vi "Test Add Parent UID To Child Node.vi"(8 "error in (no error)":errorcluster) -> (0 "error out":errorcluster)   [LabVIEW 2017, in "Unit Tests.lvlib"]
uses:
  Unit Tests.lvlib
  source/Browser Core/Server Classes/Base Tree/Base Tree.lvclass
  source/Browser Core/Node Classes/Generic Node/Generic Node.lvclass
  source/Browser Core/Server Classes/Base Tree/Base Tree.lvclass/Base Tree.ctl
  source/Browser Core/Node Classes/Generic Node/Generic Node.lvclass/Generic Node.ctl
  <vilib>/addons/_JKI Toolkits/Caraya/classes/Test/Test.lvclass
  <vilib>/addons/_JKI Toolkits/Caraya/classes/Assert/Assert.lvclass
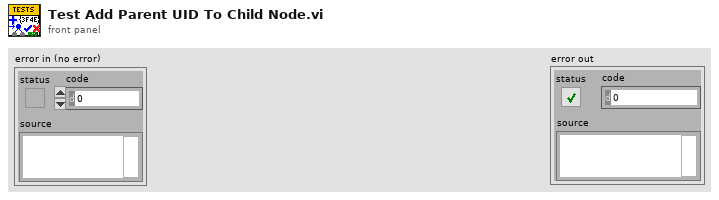
[diagram p1: front panel]
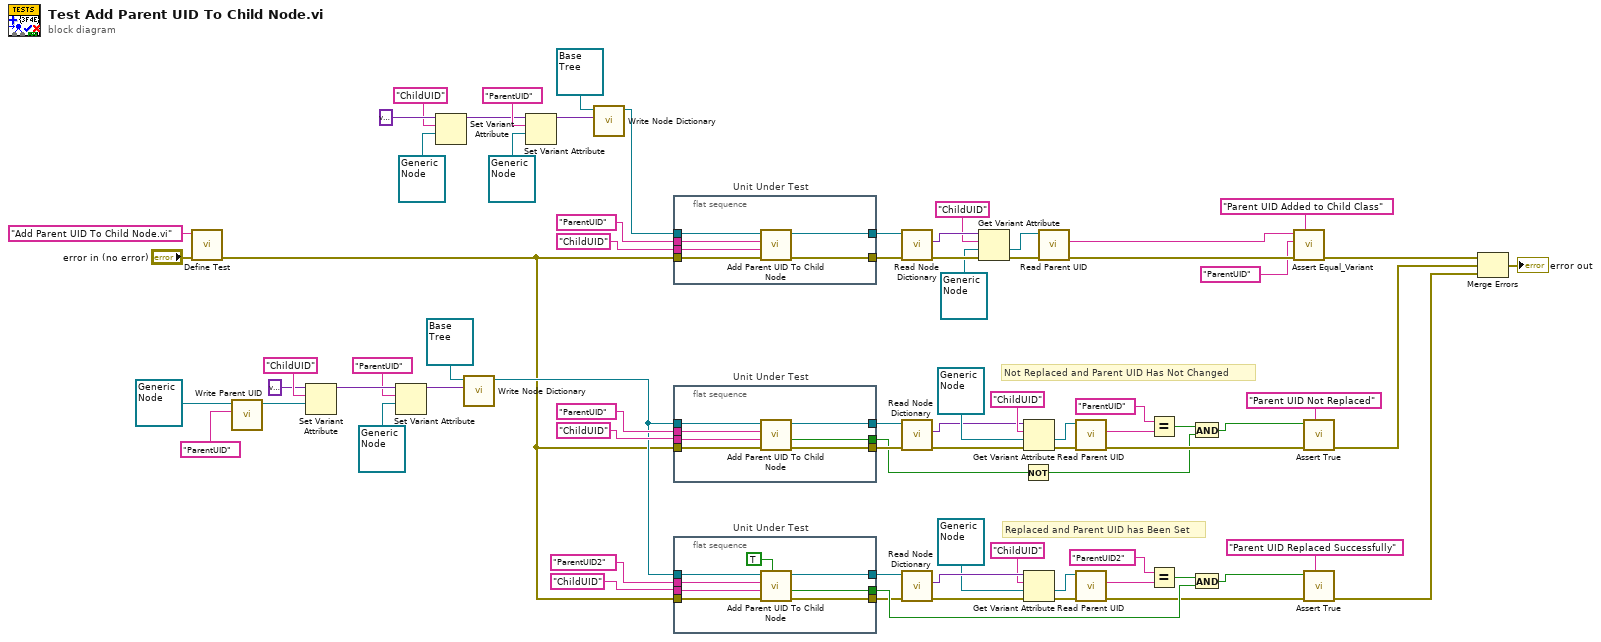
[diagram p0: block diagram]
diagram:
  # "Replaced and Parent UID has Been Set"
  # "Not Replaced and Parent UID Has Not Changed"
  n1 = call <vilib>:"Define Test.vi"("error in (no error)"="error in (no error)", "Label (VI Title)"="Add Parent UID To Child Node.vi") -> ("error out"=w3:errorcluster)  [unwired: 9 in]
  n2 = call "Write Parent UID.vi"("Parent UID"="ParentUID" ("name"), "Generic Node in"=refnum<class "Generic Node.lvclass"> refnum ("Browser Core.lvlib:Generic Node.lvclass")) -> ("Generic Node out"=w28:refnum<class "Generic Node.lvclass">)  [unwired: 8 in, 1 out]
  n3 = Set Variant Attribute(Variant=variant ("variant"), name="ChildUID", value=w28) -> (Variant out=w36:variant)  [unwired: 1 in, 2 out]
  n4 = Set Variant Attribute(Variant=w36, name="ParentUID", value=refnum<class "Generic Node.lvclass"> refnum ("Browser Core.lvlib:Generic Node.lvclass")) -> (Variant out=w37:variant)  [unwired: 1 in, 2 out]
  n5 = Set Variant Attribute(Variant=variant ("variant"), name="ChildUID", value=refnum<class "Generic Node.lvclass"> refnum ("Browser Core.lvlib:Generic Node.lvclass")) -> (Variant out=w68:variant)  [unwired: 1 in, 2 out]
  n6 = call "Write Node Dictionary.vi"("Node Dictionary"=w37, "Base Tree in"=refnum<class "Base Tree.lvclass"> refnum) -> ("Base Tree out"=w4:refnum<class "Base Tree.lvclass">)  [unwired: 8 in, 1 out]
  n7 = Set Variant Attribute(Variant=w68, name="ParentUID", value=refnum<class "Generic Node.lvclass"> refnum ("Browser Core.lvlib:Generic Node.lvclass")) -> (Variant out=w67:variant)  [unwired: 1 in, 2 out]
  n8 = call "Write Node Dictionary.vi"("Node Dictionary"=w67, "Base Tree in"=refnum<class "Base Tree.lvclass"> refnum) -> ("Base Tree out"=w40:refnum<class "Base Tree.lvclass">)  [unwired: 8 in, 1 out]
  n9 = flat-sequence "Unit Under Test" {
    tunnel: w3 -> [w82]
    tunnel: w40 -> [w81]
    tunnel: "ParentUID" ("name") -> [w80]
    tunnel: "ChildUID" ("name") -> [w79]
    tunnel: [w78] -> w64
    tunnel: [w77] -> w63
    frame #0 {
      n10 = call "Add Parent UID To Child Node.vi"("error in (no error)"=w82, "Child UID"=w79, "Parent UID"=w80, "Base Tree in"=w81) -> ("error out"=w78:errorcluster, "Base Tree out"=w77:refnum<class "Base Tree.lvclass">)  [unwired: 5 in, 1 out]
    }
  }
  n11 = flat-sequence "Unit Under Test" {
    tunnel: w3 -> [w89]
    tunnel: w4 -> [w88]
    tunnel: "ParentUID" ("name") -> [w87]
    tunnel: "ChildUID" ("name") -> [w86]
    tunnel: [w85] -> w41
    tunnel: [w84] -> w42
    tunnel: [w83] -> w23
    frame #0 {
      n12 = call "Add Parent UID To Child Node.vi"("error in (no error)"=w89, "Child UID"=w86, "Parent UID"=w87, "Base Tree in"=w88) -> ("error out"=w85:errorcluster, "Replaced?"=w83:bool, "Base Tree out"=w84:refnum<class "Base Tree.lvclass">)  [unwired: 5 in]
    }
  }
  n13 = flat-sequence "Unit Under Test" {
    tunnel: w3 -> [w97]
    tunnel: w4 -> [w96]
    tunnel: "ParentUID2" ("name") -> [w95]
    tunnel: "ChildUID" ("name") -> [w94]
    tunnel: [w93] -> w14
    tunnel: [w92] -> w13
    tunnel: [w91] -> w21
    frame #0 {
      n14 = call "Add Parent UID To Child Node.vi"("Replace? (F)"=TRUE, "error in (no error)"=w97, "Child UID"=w94, "Parent UID"=w95, "Base Tree in"=w96) -> ("error out"=w93:errorcluster, "Replaced?"=w91:bool, "Base Tree out"=w92:refnum<class "Base Tree.lvclass">)  [unwired: 4 in]
    }
  }
  n15 = call "Read Node Dictionary.vi"("error in (no error)"=w64, "Base Tree in"=w63) -> ("error out"=w62:errorcluster, "Node Dictionary"=w61:variant)  [unwired: 7 in, 1 out]
  n16 = call "Read Node Dictionary.vi"("error in (no error)"=w41, "Base Tree in"=w42) -> ("error out"=w43:errorcluster, "Node Dictionary"=w44:variant)  [unwired: 7 in, 1 out]
  n17 = call "Read Node Dictionary.vi"("error in (no error)"=w14, "Base Tree in"=w13) -> ("error out"=w12:errorcluster, "Node Dictionary"=w11:variant)  [unwired: 7 in, 1 out]
  n18 = Get Variant Attribute(Variant=w61, name="ChildUID", default value (empty Variant)=refnum<class "Generic Node.lvclass"> refnum ("Browser Core.lvlib:Generic Node.lvclass"), error in=w62) -> (value=w57:refnum<class "Generic Node.lvclass">, error out=w58:errorcluster)  [unwired: 2 out]
  n19 = Not(x=w23) -> (.not. x?=w22:bool)
  n20 = Get Variant Attribute(Variant=w44, name="ChildUID", default value (empty Variant)=refnum<class "Generic Node.lvclass"> refnum ("Browser Core.lvlib:Generic Node.lvclass"), error in=w43) -> (value=w48:refnum<class "Generic Node.lvclass">, error out=w47:errorcluster)  [unwired: 2 out]
  n21 = Get Variant Attribute(Variant=w11, name="ChildUID", default value (empty Variant)=refnum<class "Generic Node.lvclass"> refnum ("Browser Core.lvlib:Generic Node.lvclass"), error in=w12) -> (value=w7:refnum<class "Generic Node.lvclass">, error out=w8:errorcluster)  [unwired: 2 out]
  n22 = call "Read Parent UID.vi"("error in (no error)"=w58, "Generic Node in"=w57) -> ("error out"=w56:errorcluster, "Parent UID"=w54:string)  [unwired: 7 in, 1 out]
  n23 = call "Read Parent UID.vi"("error in (no error)"=w47, "Generic Node in"=w48) -> ("error out"=w49:errorcluster, "Parent UID"=w27:string)  [unwired: 7 in, 1 out]
  n24 = call "Read Parent UID.vi"("error in (no error)"=w8, "Generic Node in"=w7) -> ("error out"=w6:errorcluster, "Parent UID"=w17:string)  [unwired: 7 in, 1 out]
  n25 = Equal?(x="ParentUID" ("name"), y=w27) -> (x = y?=w25:bool)
  n26 = Equal?(x="ParentUID2" ("name"), y=w17) -> (x = y?=w19:bool)
  n27 = And(x=w25, y=w22) -> (x .and. y?=w24:bool)
  n28 = And(x=w19, y=w21) -> (x .and. y?=w20:bool)
  n29 = call <vilib>:"Assert Equal_Variant.vi"("Label"="Parent UID Added to Child Class", "error in (no error)"=w56, "Y"="ParentUID" ("name"), "X"=w54) -> ("error out"=w52:errorcluster)  [unwired: 7 in]
  n30 = call <vilib>:"Assert True.vi"("Label"="Parent UID Not Replaced", "error in (no error)"=w49, "True?"=w24) -> ("error out"=w2:errorcluster)  [unwired: 8 in]
  n31 = call <vilib>:"Assert True.vi"("Label"="Parent UID Replaced Successfully", "error in (no error)"=w6, "True?"=w20) -> ("error out"=w1:errorcluster)  [unwired: 8 in]
  n32 = Merge Errors(w52, w2, w1) -> (→"error out":errorcluster)
